vi "AnalysisPannel.vi"() -> ()   [LabVIEW 2012]
panel:
  out "MousePos":cluster{"X":dbl, "Y":dbl}
  in  "停止":bool
  out "Sigma":cluster{"StdX":dbl, "StdY":dbl}(graph)
  out "Pos":cluster{"PosX":dbl, "PosY":dbl}(graph)
  out "Amp":dbl(graph)
  out "强度图":u16[][](graph)
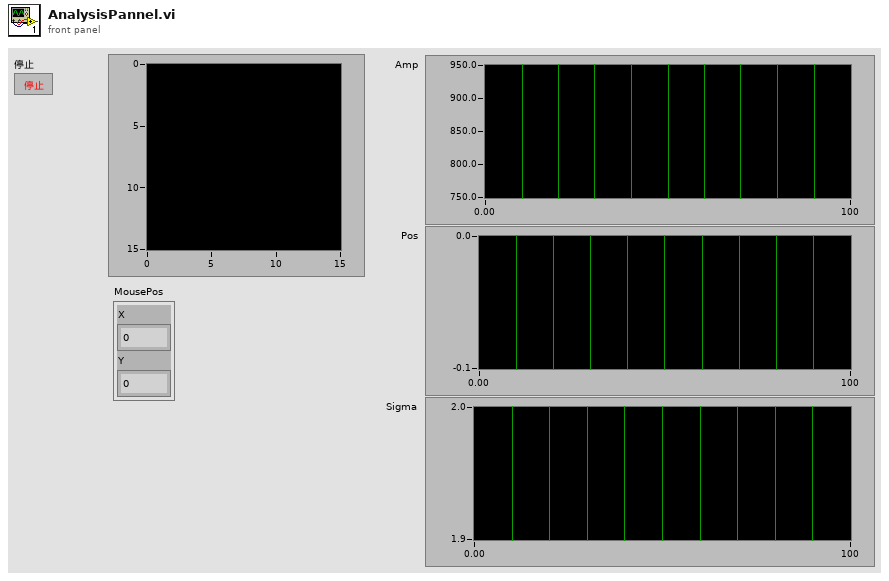
[diagram p1: front panel]
types:
  T1 = cluster{"Position":cluster{"X":dbl, "Y":dbl}, "DoubleClick":bool}
  T2 = cluster{"image":i16[][], "x_start":u32, "x_end":u32, "y_start":u32, "y_end":u32, "ImageCnt":u32, "subImage":u16[][]}
  T3 = cluster{"Amp":dbl, "PosX":dbl, "PosY":dbl, "StdX":dbl, "StdY":dbl, "Bkg":dbl, "Steps":i32, "time":dbl}
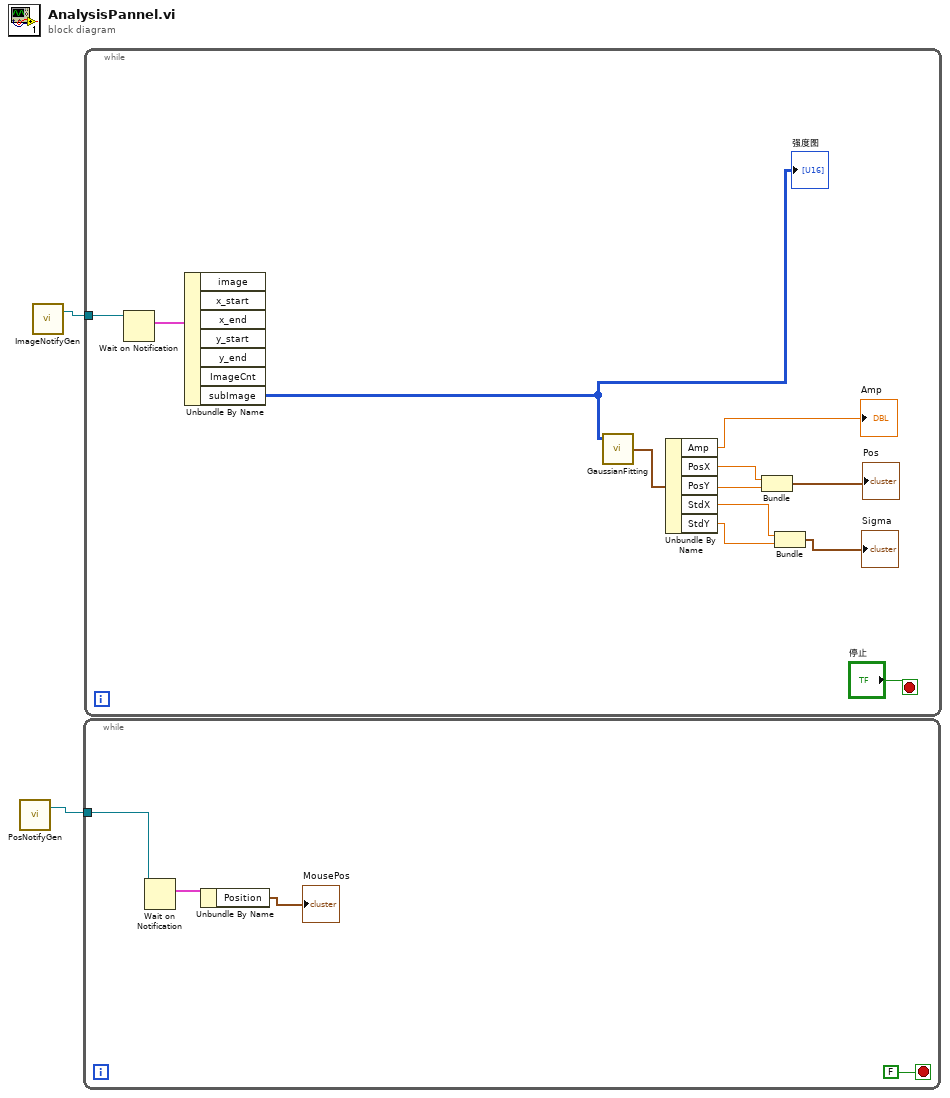
[diagram p0: block diagram]
diagram:
  n1 = call "PosNotifyGen.vi"() -> ("NotifyRef"=w1:refnum<notifier>)  [unwired: 2 in, 1 out]
  n2 = call "ImageNotifyGen.vi"() -> ("ImageNotifyRef"=w2:refnum<notifier>)  [unwired: 2 in, 1 out]
  n3 = while {
    tunnel: w1 -> [w6]
    stop <- FALSE stop-if-true
    n4 = Wait on Notification(notifier=w6) -> (notification=w4:T1)  [unwired: 3 in, 3 out]
    n5 = Unbundle By Name(w4) -> ("Position"=→"MousePos":cluster{"X":dbl, "Y":dbl})
  }
  n6 = while {
    tunnel: w2 -> [w18]
    stop <- "停止" stop-if-true
    n7 = Wait on Notification(notifier=w18) -> (notification=w17:T2)  [unwired: 3 in, 3 out]
    n8 = Unbundle By Name(w17) -> ("subImage"=w13:u16[][])  [unwired: 6 out]
    "强度图" <- w13
    n9 = call "GaussianFitting.vi"("数组"=w13) -> ("Result"=w16:T3)  [unwired: 2 in]
    n10 = Unbundle By Name(w16) -> ("Amp"=→"Amp":dbl, "PosX"=w12:dbl, "PosY"=w11:dbl, "StdX"=w9:dbl, "StdY"=w8:dbl)
    n11 = Bundle("PosX"=w12, "PosY"=w11) -> (→"Pos":cluster{"PosX":dbl, "PosY":dbl})  [unwired: 1 in]
    n12 = Bundle("StdX"=w9, "StdY"=w8) -> (→"Sigma":cluster{"StdX":dbl, "StdY":dbl})  [unwired: 1 in]
  }
